vi "Read SQLite Connection.vi"(8 "error in (no error)":errorcluster, 11 "SQLite_API in":refnum<class "SQLite_API.lvclass">) -> (0 "error out":errorcluster, 2 "SQLite.lvlib:Connection":refnum<class "Connection.lvclass">, 3 "SQLite_API out":refnum<class "SQLite_API.lvclass">)   [LabVIEW 2021, in "SQLite_API.lvclass"]
uses:
  <userlib>/John_Lib/DataBase/SQLite_API/SQLite_API.lvclass
  <userlib>/John_Lib/DataBase/SQLite_API/SQLite_API.lvclass/SQLite_API.ctl
  <vilib>/drjdpowell/SQLite Library/SQL Connection/Connection.lvclass
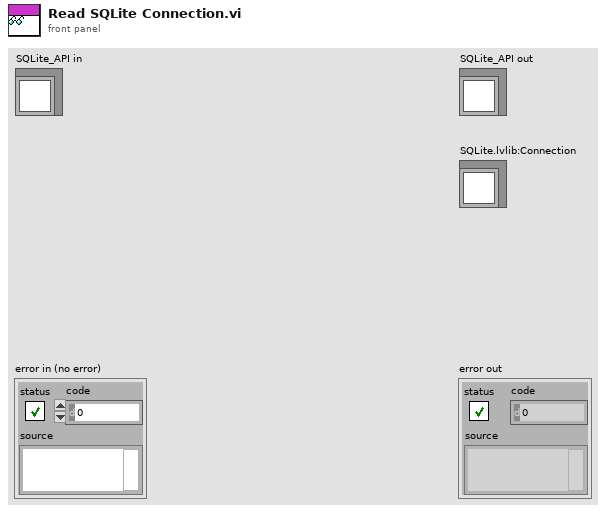
[diagram p1: front panel]
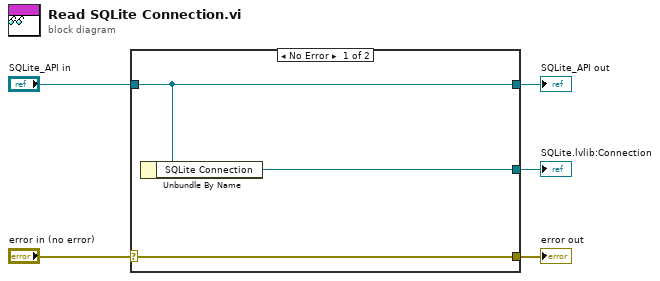
[diagram p0: block diagram]
diagram:
  n1 = case shown="No Error" "error in (no error)" {
    selector: "error in (no error)" -> [w8 w9]
    tunnel: [w8 w9] -> w4
    tunnel: [w7 w10] -> w2
    tunnel: "SQLite_API in" -> [w7 w10]
    tunnel: [w6 _] -> w1
    frame No Error {
      n2 = Unbundle By Name(w7) -> ("SQLite Connection"=w6:refnum<class "Connection.lvclass">)
    }
    frame Error {
    }
  }
  "error out" <- w4
  "SQLite_API out" <- w2
  "SQLite.lvlib:Connection" <- w1
